vi "Audio_Transformation_Setted_Frequency_v007.vi"() -> ()   [LabVIEW 2019]
uses:
  <vilib>/addons/_Advanced Signal Processing/NI_AdvSigProcTFA.lvlib
  <vilib>/sound2/lvsound2.llb/Sound Data Format.ctl
  <vilib>/sound2/lvsound2.llb/Sound Input Read (DBL).vi
  <vilib>/addons/Time Frequency Analysis/Transform.llb/TFA Online Gabor Transform (Real).vi
panel:
  out "u(t)":T1(graph)
  out "V(t)":T1(graph)
  out "Noise Speech":dbl[](graph)
  in  "Address selector":i32[](array[numeric])
  in  "Neuron Type":T2(ring)
  out "max index(es)":i32
  out "max value":dbl
  out "Waveform Graph":dbl[](graph)
  out "Magnitude of Gabor Coefficients":dbl[][](graph)
  in  "Stop":bool
  # "Step two : Graph of the amplitude of the Gabor coefficient of the different bins"
  # "Step three : Spike Response of the neurons"
  # "Step one: Sound recorded from the computer"
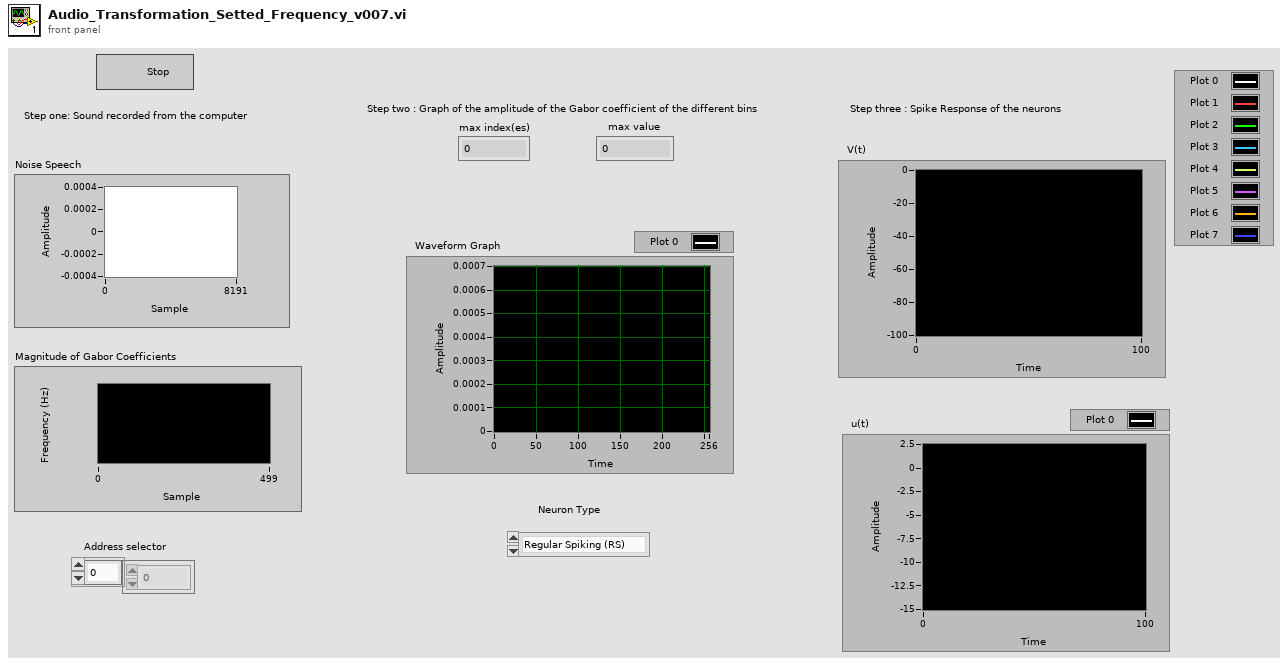
[diagram p1: front panel]
types:
  T1 = cluster{"[0]":dbl, "[1]":dbl, "[2]":dbl, "[3]":dbl, "[4]":dbl, "[5]":dbl, "[6]":dbl, "[7]":dbl}
  T2 = enum16{"Regular Spiking (RS)", "Intrinsically Bursting (IB)", "Chattering (CH)", "Fast Spiking (FS)", "Thalamo-Cortical 1 (TC1)", "Thalamo-Cortical 2 (TC2)", "Resonator (RZ)", "Low-Threshold Spiking (LTS)"}
  T3 = typedef "Sound Data Format.ctl" = cluster{"sample rate (S/s)":dbl, "number of channels":i32, "bits per sample":i32}
  T4 = cluster{"analysis window":dbl[], "dM (time steps)":i32, "N (frequency bins)":i32}
  T5 = typedef "Sound Input Task ID.ctl" = u32
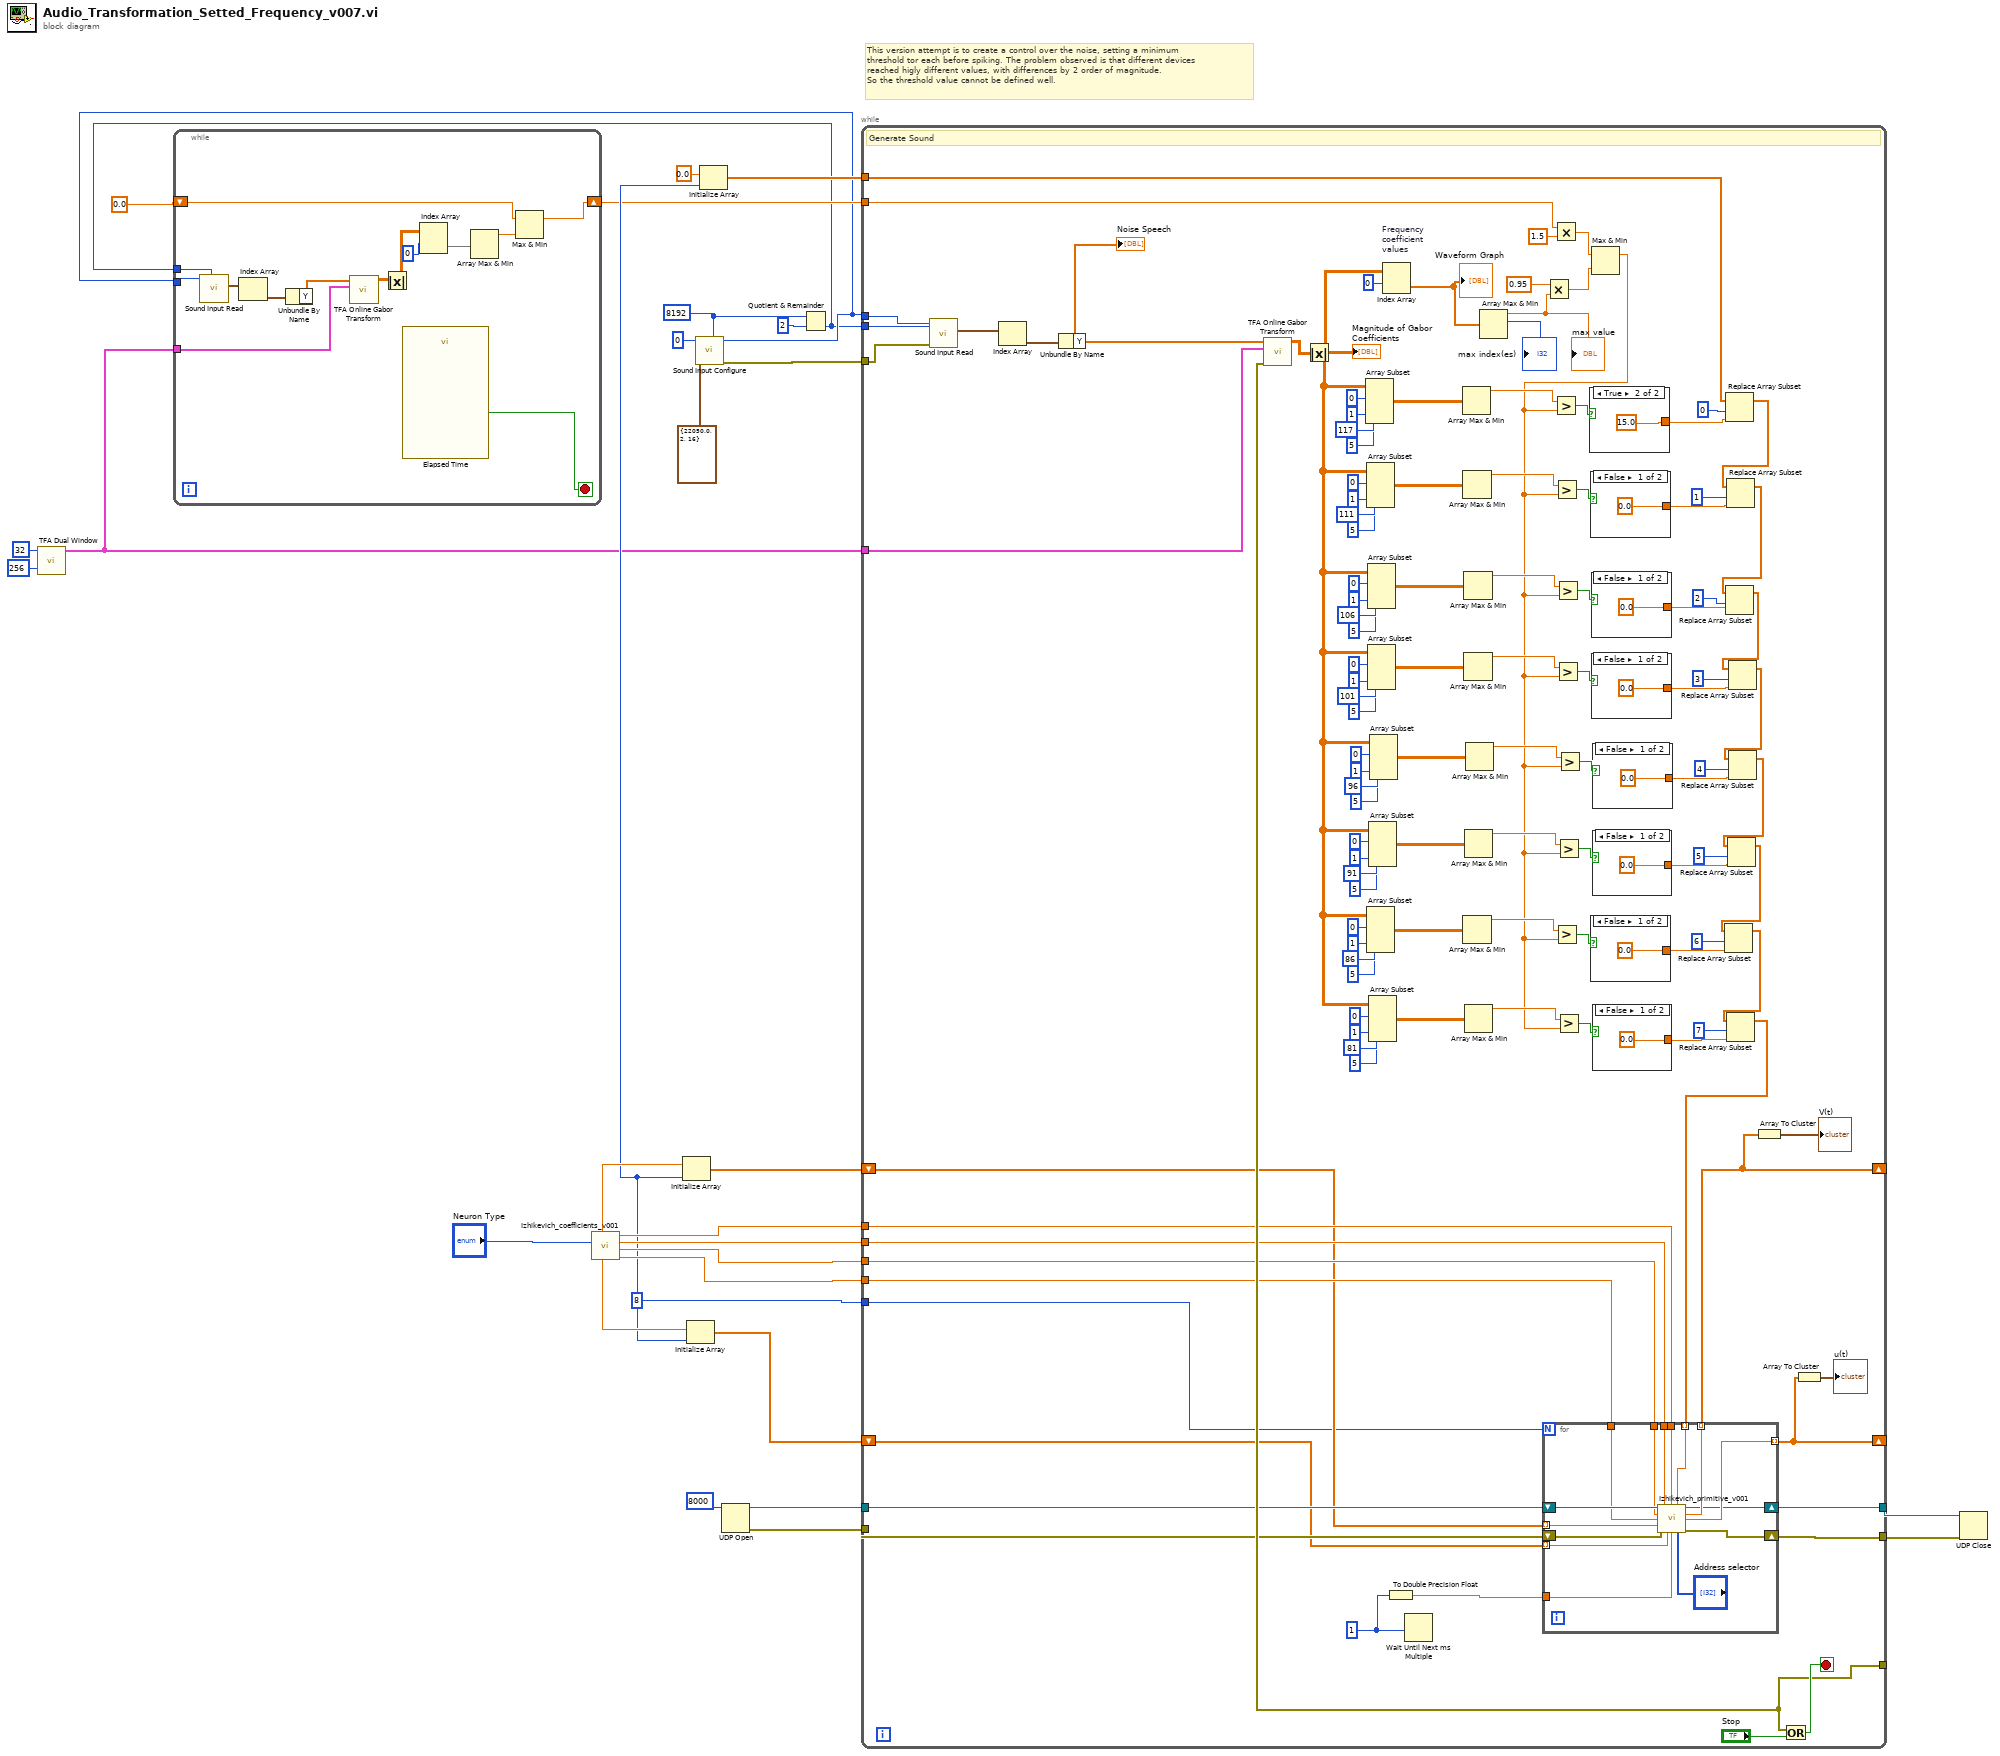
[diagram p0: block diagram]
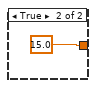
[diagram p2: hidden frame]
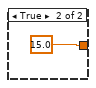
[diagram p3: hidden frame]
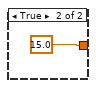
[diagram p4: hidden frame]
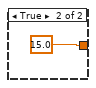
[diagram p5: hidden frame]
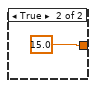
[diagram p6: hidden frame]
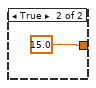
[diagram p7: hidden frame]
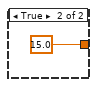
[diagram p8: hidden frame]
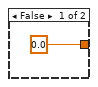
[diagram p9: hidden frame]
diagram:
  w8 = 8
  w15 = 8192 ("number of samples/ch")
  # "This version attempt is to create a control over the noise, setting a minimum\nthreshold tor each before spiking. The problem observed is that different devices\nreached higly different values, with differences by 2 order of magnitude.\nSo the threshold value cannot be defined well."
  n1 = call <vilib>:"TFA Dual Window.vi"("N (frequency bins)"=256, "dM (time steps)"=32) -> ("analysis info"=w5:T4)  [unwired: 7 in, 2 out]
  n2 = call "Izhikevich_coefficients_v001.vi"("Neuron Type"="Neuron Type") -> ("d"=w23:dbl, "c"=w24:dbl, "b"=w25:dbl, "a"=w26:dbl, "u0"=w10:dbl, "v0"=w12:dbl)  [unwired: 3 in]
  n3 = Initialize Array(w12, w8) -> (w11:dbl[])
  n4 = Initialize Array(w10, w8) -> (w9:dbl[])
  n5 = call <vilib>:"Sound Input Configure.vi"("number of samples/ch"=w15, "sound format"=T3 {"sample rate (S/s)"=22050.0, "number of channels"=2, "bits per sample"=16}, "device ID"=u32 0) -> ("error out"=w13:errorcluster, "task ID"=w2:T5)  [unwired: 7 in]
  n6 = Initialize Array(0.0 ("element"), w8) -> (w6:dbl[])
  n7 = UDP Open(11:u16 8000 ("port")) -> (port=w21:refnum<k16>, 0:w20:errorcluster)  [unwired: 4 in, 1 out]
  n8 = Quotient & Remainder(x=w15, y=2) -> (floor(x/y)=w1:i32)  [unwired: 1 out]
  n9 = while {
    tunnel: w5 -> [w41]
    shift-right: [w33] -> w3
    shift-left: 0.0 -> [w34]
    tunnel: w2 -> [w31]
    tunnel: w1 -> [w30]
    stop <- w32 stop-if-true
    n10 = call-poly <vilib>:"Sound Input Read.vi"("number of samples/ch"=w30, "task ID"=w31) -> ("data"=w42:waveform(dbl)[])  [unwired: 7 in, 2 out]
    n11 = Index Array(array=w42) -> (element=w43:waveform(dbl))  [unwired: 1 in]
    n12 = Unbundle By Name(w43) -> ("Y"=w40:dbl[])
    n13 = call-poly <vilib>:"TFA Online Gabor Transform.vi"("transform info"=w41, "signal"=w40) -> ("Gabor coef"=w39:cdb[][])  [unwired: 7 in, 2 out]
    n14 = Absolute Value(x=w39) -> (abs(x)=w37:dbl[][])
    n15 = call "Elapsed Time"() -> ("Time has Elapsed"=w32:bool)  [unwired: 12 in, 7 out]
    n16 = Index Array(array=w37, index (row)=0) -> (element=w36:dbl[])  [unwired: 1 in]
    n17 = Array Max & Min(array=w36) -> (max value=w35:dbl)  [unwired: 3 out]
    n18 = Max & Min(x=w34, y=w35) -> (max(x,y)=w33:dbl)  [unwired: 1 out]
  }
  n19 = while {
    tunnel: [w156] -> _
    tunnel: w5 -> [w161]
    shift-right: [w54] -> _
    shift-left: w11 -> [w145]
    shift-right: [w52] -> _
    shift-left: w9 -> [w144]
    tunnel: w26 -> [w155]
    tunnel: w25 -> [w154]
    tunnel: w24 -> [w152]
    tunnel: w23 -> [w151]
    tunnel: w21 -> [w153]
    tunnel: w20 -> [w150]
    tunnel: [w147] -> w19
    tunnel: [w146] -> w18
    tunnel: w2 -> [w142]
    tunnel: w13 -> [w141]
    tunnel: w1 -> [w143]
    tunnel: w8 -> [w137]
    tunnel: w6 -> [w109]
    tunnel: w3 -> [w48]
    stop <- w162 stop-if-true
    w149 = u32 1 ("millisecond multiple")
    # "Generate Sound"
    n20 = call-poly <vilib>:"Sound Input Read.vi"("number of samples/ch"=w143, "error in (no error)"=w141, "task ID"=w142) -> ("data"=w139:waveform(dbl)[])  [unwired: 6 in, 2 out]
    n21 = Index Array(array=w139) -> (element=w140:waveform(dbl))  [unwired: 1 in]
    n22 = Unbundle By Name(w140) -> ("Y"=w138:dbl[])
    "Noise Speech" <- w138
    n23 = call-poly <vilib>:"TFA Online Gabor Transform.vi"("transform info"=w161, "signal"=w138) -> ("error out"=w156:errorcluster, "Gabor coef"=w160:cdb[][])  [unwired: 7 in, 1 out]
    n24 = Absolute Value(x=w160) -> (abs(x)=w57:dbl[][])
    "Magnitude of Gabor Coefficients" <- w57
    n25 = Array Subset(array=w57, index (row)=0 ("index"), length (row)=1 ("length"), index (col)=117 ("index"), length (col)=5 ("length")) -> (w132:dbl[][])
    n26 = Array Subset(array=w57, index (row)=0 ("index"), length (row)=1 ("length"), index (col)=111 ("index"), length (col)=5 ("length")) -> (w125:dbl[][])
    n27 = Array Subset(array=w57, index (row)=0 ("index"), length (row)=1 ("length"), index (col)=86 ("index"), length (col)=5 ("length")) -> (w72:dbl[][])
    n28 = Array Subset(array=w57, index (row)=0 ("index"), length (row)=1 ("length"), index (col)=106 ("index"), length (col)=5 ("length")) -> (w114:dbl[][])
    n29 = Array Subset(array=w57, index (row)=0 ("index"), length (row)=1 ("length"), index (col)=101 ("index"), length (col)=5 ("length")) -> (w102:dbl[][])
    n30 = Array Subset(array=w57, index (row)=0 ("index"), length (row)=1 ("length"), index (col)=91 ("index"), length (col)=5 ("length")) -> (w82:dbl[][])
    n31 = Array Subset(array=w57, index (row)=0 ("index"), length (row)=1 ("length"), index (col)=81 ("index"), length (col)=5 ("length")) -> (w62:dbl[][])
    n32 = Array Subset(array=w57, index (row)=0 ("index"), length (row)=1 ("length"), index (col)=96 ("index"), length (col)=5 ("length")) -> (w92:dbl[][])
    n33 = Index Array "Frequency \ncoefficient \nvalues"(array=w57, index (row)=0) -> (element=w158:dbl[])  [unwired: 1 in]
    "Waveform Graph" <- w158
    n34 = To Double Precision Float(number=w149) -> (double precision float=w148:dbl)
    n35 = Wait Until Next ms Multiple(millisecond multiple=w149) -> ()  [unwired: 1 out]
    n36 = Array Max & Min(array=w132) -> (max value=w131:dbl)  [unwired: 3 out]
    n37 = Array Max & Min(array=w125) -> (max value=w124:dbl)  [unwired: 3 out]
    n38 = Array Max & Min(array=w72) -> (max value=w71:dbl)  [unwired: 3 out]
    n39 = Array Max & Min(array=w114) -> (max value=w113:dbl)  [unwired: 3 out]
    n40 = Array Max & Min(array=w102) -> (max value=w101:dbl)  [unwired: 3 out]
    n41 = Array Max & Min(array=w82) -> (max value=w81:dbl)  [unwired: 3 out]
    n42 = Array Max & Min(array=w62) -> (max value=w61:dbl)  [unwired: 3 out]
    n43 = Array Max & Min(array=w92) -> (max value=w91:dbl)  [unwired: 3 out]
    n44 = Array Max & Min(array=w158) -> (max value=w45:dbl, max index (indices)=→"max index(es)":i32)  [unwired: 2 out]
    "max value" <- w45
    n45 = Multiply(x=0.95 ("y"), y=w45) -> (x*y=w46:dbl)
    n46 = Multiply(x=w48, y=1.5) -> (x*y=w47:dbl)
    n47 = Max & Min(x=w47, y=w46) -> (max(x,y)=w50:dbl)  [unwired: 1 out]
    n48 = Greater?(x=w131, y=w50) -> (0:w130:bool)
    n49 = Greater?(x=w124, y=w50) -> (0:w123:bool)
    n50 = Greater?(x=w71, y=w50) -> (0:w70:bool)
    n51 = Greater?(x=w113, y=w50) -> (0:w112:bool)
    n52 = Greater?(x=w101, y=w50) -> (0:w100:bool)
    n53 = Greater?(x=w81, y=w50) -> (0:w80:bool)
    n54 = Greater?(x=w61, y=w50) -> (0:w60:bool)
    n55 = Greater?(x=w91, y=w50) -> (0:w90:bool)
    n56 = case shown="True" w130 {
      tunnel: [0.0 15.0] -> w122
      frame False {
      }
      frame True {
      }
    }
    n57 = case shown="False" w123 {
      tunnel: [0.0 15.0] -> w119
      frame False {
      }
      frame True {
      }
    }
    n58 = case shown="False" w70 {
      tunnel: [0.0 15.0] -> w68
      frame False {
      }
      frame True {
      }
    }
    n59 = case shown="False" w112 {
      tunnel: [0.0 15.0] -> w110
      frame False {
      }
      frame True {
      }
    }
    n60 = case shown="False" w100 {
      tunnel: [0.0 15.0] -> w98
      frame False {
      }
      frame True {
      }
    }
    n61 = case shown="False" w80 {
      tunnel: [0.0 15.0] -> w78
      frame False {
      }
      frame True {
      }
    }
    n62 = case shown="False" w60 {
      tunnel: [0.0 15.0] -> w58
      frame False {
      }
      frame True {
      }
    }
    n63 = case shown="False" w90 {
      tunnel: [0.0 15.0] -> w88
      frame False {
      }
      frame True {
      }
    }
    n64 = Replace Array Subset(array=w109, new element=w122, index=0) -> (w108:dbl[])
    n65 = Replace Array Subset(array=w108, new element=w119, index=1) -> (w107:dbl[])
    n66 = Replace Array Subset(array=w107, new element=w110, index=2) -> (w97:dbl[])
    n67 = Replace Array Subset(array=w97, new element=w98, index=3) -> (w87:dbl[])
    n68 = Replace Array Subset(array=w87, new element=w88, index=4) -> (w77:dbl[])
    n69 = Replace Array Subset(array=w77, new element=w78, index=5) -> (w67:dbl[])
    n70 = Replace Array Subset(array=w67, new element=w68, index=6) -> (w56:dbl[])
    n71 = Replace Array Subset(array=w56, new element=w58, index=7) -> (w55:dbl[])
    n72 = for {
      N: w137 -> [_]
      tunnel: w155 -> [w194]
      tunnel: w154 -> [w193]
      tunnel: w152 -> [w191]
      tunnel: w151 -> [w190]
      tunnel: w148 -> [w187]
      tunnel: [w186] -> w54 mode=indexing
      tunnel: [w185] -> w52 mode=indexing
      tunnel: w145 -> [w182] mode=indexing
      tunnel: w144 -> [w181] mode=indexing
      shift-right: [w183] -> w146
      shift-left: w153 -> [w192]
      shift-right: [w184] -> w147
      shift-left: w150 -> [w189]
      tunnel: w55 -> [w180] mode=indexing
      n73 = call "Izhikevich_primitive_v001.vi"("UDP Network Connection in"=w192, "b"=w193, "a"=w194, "I"=w180, "c"=w191, "d"=w190, "v(t)"=w182, "error in (no error)"=w189, "u(t)"=w181, "Numeric"=w187, "Address selector"="Address selector") -> ("UDP Network Connection out"=w183:refnum<k16>, "v(t+dt)"=w186:dbl, "u(t+dt)"=w185:dbl, "error out"=w184:errorcluster)  [unwired: 1 in]
    }
    n74 = Array To Cluster(array=w54) -> (cluster=→"V(t)":T1)
    n75 = Or(x=w156, y="Stop") -> (x .or. y?=w162:bool)
    n76 = Array To Cluster(array=w52) -> (cluster=→"u(t)":T1)
  }
  n77 = UDP Close(connection ID=w18, 8:w19) -> ()  [unwired: 2 out]
